vi "Set DC Voltage.vi"(8 "error in":errorcluster, 10 "Voltage":dbl format="%#_g V", 11 "PXI-5441 in":refnum<class "Fgen PXI.lvclass">) -> (0 "error out":errorcluster, 3 "PXI-5441 out":refnum<class "Fgen PXI.lvclass">)   [LabVIEW 2023, in "HAL.lvlib" / "Fgen PXI.lvlib" / "Fgen PXI.lvclass"]
uses:
  Fgen PXI.lvclass
  Fgen PXI.lvclass/Fgen PXI.ctl
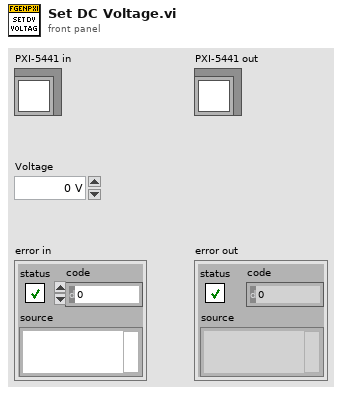
[diagram p1: front panel]
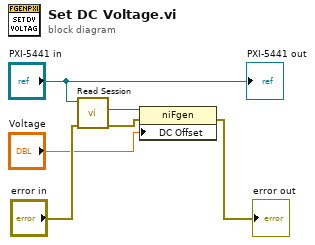
[diagram p0: block diagram]
diagram:
  n1 = call "Read Session.vi"("error in"="error in", "Fgen PXI in"="PXI-5441 in") -> ("error out"=w3:errorcluster, "Session"=w4:refnum<k15>)  [unwired: 7 in, 1 out]
  n2 = property class="niFgen"(reference=w4, error in=w3, "DC Offset"="Voltage") -> (error out=→"error out":errorcluster)  [unwired: 1 out]
  "PXI-5441 out" <- "PXI-5441 in"
